vi "Main.vi"() -> ()   [LabVIEW 2016, in "Utilities.lvlib" / "Joystick.lvlib"]
uses:
  Joystick/Joystick.lvlib
  Joystick/Controls/Speed Scale.ctl
  Joystick/Controls/Up.ctl
  Joystick/Controls/Right.ctl
  Joystick/Controls/Left.ctl
  Joystick/Controls/Down.ctl
  Drivers/Agilis/AgilisCmdLib Refnum.ctl
  Drivers/Agilis/Jog Mode.ctl
  Support VIs/Message Queue/Enqueue Message (Multiple).vi
  Support VIs/Message Queue/Enqueue Message (Single).vi
  Support VIs/Message Queue/Message Queue.lvlib
  Drivers/Agilis/Agilis.lvlib
  C:/Users/MyUser/Desktop/Trace Grabber/Drivers/Agilis/AgilisCmdLib.dll
  Drivers/Agilis/AgilisCmdLib.dll
panel:
  in  "Z":cluster{"Z-":T1, "Z+":T2}
  in  "XY":cluster{"Y+":T3, "X+":T2, "X-":T1, "Y-":T4}
  in  "Speed":T5 scale=1.0..4.0
  out "Z steps":i32
  out "Y Steps":i32
  out "X steps":i32
  # "X"
  # "steps"
  # "Y"
  # "steps"
  # "Z"
  # "steps"
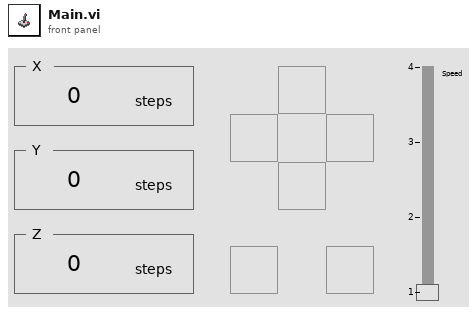
[diagram p1: front panel]
types:
  T1 = typedef "Utilities.lvlib/Joystick.lvlib/Left.ctl" = bool
  T2 = typedef "Utilities.lvlib/Joystick.lvlib/Right.ctl" = bool
  T3 = typedef "Utilities.lvlib/Joystick.lvlib/Up.ctl" = bool
  T4 = typedef "Utilities.lvlib/Joystick.lvlib/Down.ctl" = bool
  T5 = typedef "Utilities.lvlib/Joystick.lvlib/Speed Scale.ctl" = i32
  T6 = typedef "Drivers.lvlib/Agilis.lvlib/AgilisCmdLib Refnum.ctl" = refnum<k24>
  T7 = cluster{"Handle":T6, "Speed Option":i32, "Active Axis Index":i32, "Active Axis":cluster{"Channel":i32, "Axis":i32}}
  T8 = typedef "Drivers.lvlib/Agilis.lvlib/Jog Mode.ctl" = i32
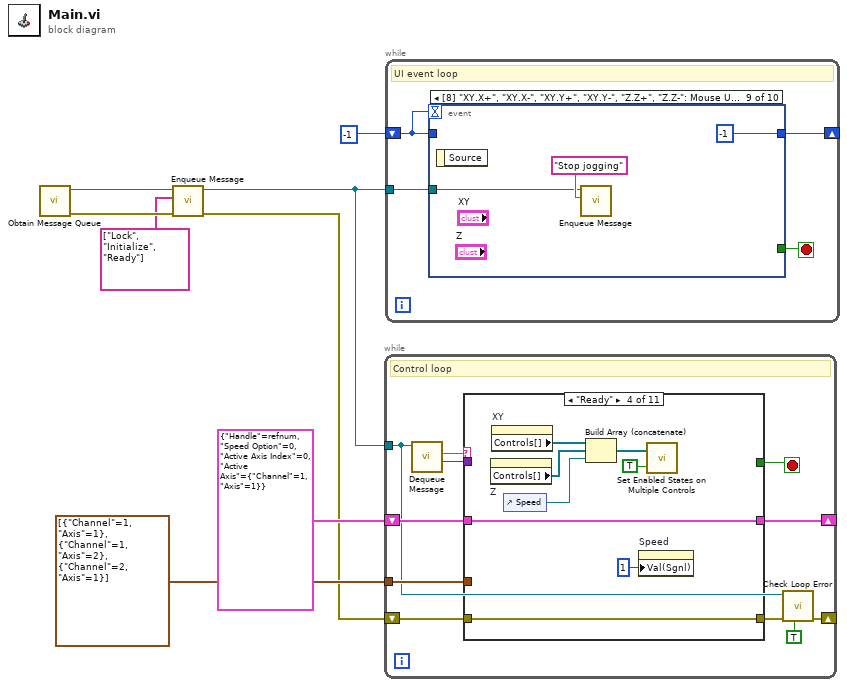
[diagram p0: block diagram]
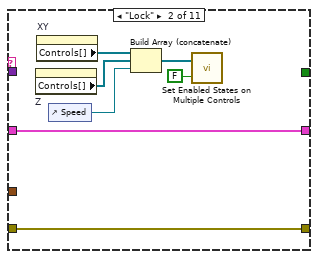
[diagram p3: hidden frame]
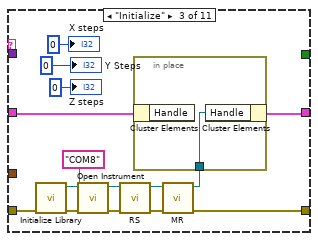
[diagram p4: hidden frame]
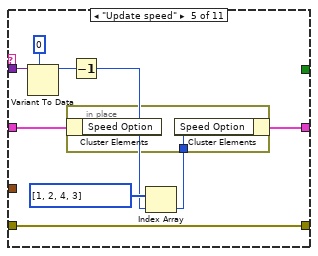
[diagram p5: hidden frame]
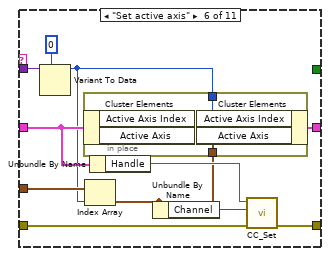
[diagram p6: hidden frame]
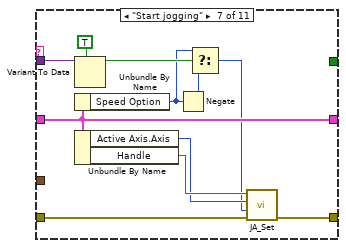
[diagram p7: hidden frame]
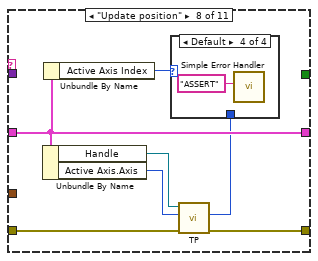
[diagram p8: hidden frame]
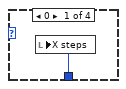
[diagram p9: hidden frame]
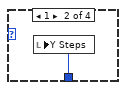
[diagram p10: hidden frame]
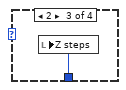
[diagram p11: hidden frame]
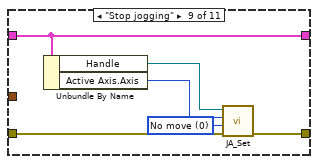
[diagram p12: hidden frame]
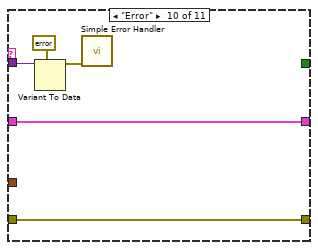
[diagram p13: hidden frame]
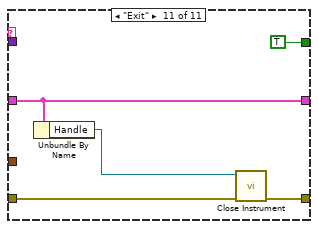
[diagram p14: hidden frame]
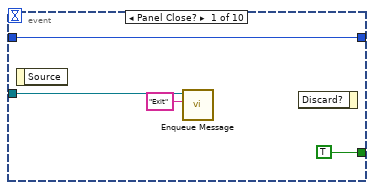
[diagram p15: hidden frame]
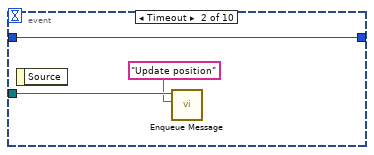
[diagram p16: hidden frame]
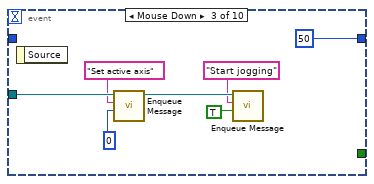
[diagram p17: hidden frame]
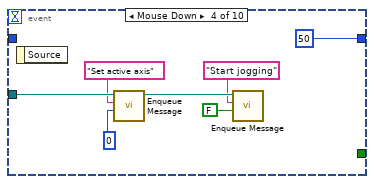
[diagram p18: hidden frame]
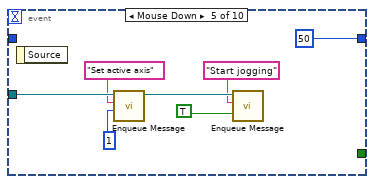
[diagram p19: hidden frame]
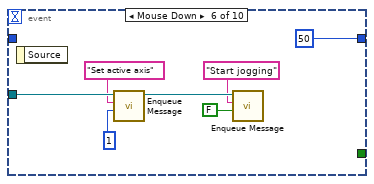
[diagram p20: hidden frame]
diagram:
  n1 = call "Obtain Message Queue.vi"() -> ("error out"=w7:errorcluster, "Message Queue out"=w8:refnum<queue>)  [unwired: 10 in]
  n2 = call-poly "Enqueue Message.vi"("error in (no error)"=w7, "States"=string[] ["Lock", "Initialize", "Ready"], "Message Queue in"=w8) -> ("error out"=w3:errorcluster, "Message Queue out"=w6:refnum<queue>)  [unwired: 7 in]
  n3 = while {
    tunnel: w6 -> [w10]
    tunnel: cluster{"Channel":i32, "Axis":i32}[] [{"Channel"=1, "Axis"=1}, {"Channel"=1, "Axis"=2}, {"Channel"=2, "Axis"=1}] -> [w18]
    shift-right: [w16] -> _
    shift-left: T7 {"Handle"=refnum, "Speed Option"=0, "Active Axis Index"=0, "Active Axis"={"Channel"=1, "Axis"=1}} -> [w15]
    shift-right: [w12] -> _
    shift-left: w3 -> [w14]
    stop <- w9 stop-if-true
    # "Control loop"
    n4 = call "Dequeue Message.vi"("Message Queue in"=w10) -> ("Data"=w17:variant, "State"=w19:string)  [unwired: 7 in, 2 out]
    n5 = case shown="\"Ready\"" w19 {
      tunnel: w18 -> [_ _ _ _ _ w70 _ _ _ _ _]
      tunnel: w15 -> [w21 w28 w40 w52 w57 w69 w81 w89 w103 w108 w113]
      tunnel: w17 -> [_ _ _ _ w60 w73 w86 _ _ w107 _]
      tunnel: [w21 w28 w39 w52 w56 w71 w81 w89 w103 w108 w113] -> w16
      tunnel: w14 -> [w20 w27 w38 w51 w53 w67 w79 w93 w99 w104 w111]
      tunnel: [w20 w27 w33 w51 w53 w66 w80 w92 w98 w104 w110] -> w13
      tunnel: [_ _ _ _ _ _ _ _ _ _ TRUE] -> w9
      frame Default {
      }
      frame "Lock" {
        n6 = property on="Z" class="Clust (strict)"() -> ("Controls[]"=w25:refnum<vi>[])  [unwired: 2 in, 2 out]
        n7 = property on="XY" class="Clust (strict)"() -> ("Controls[]"=w26:refnum<vi>[])  [unwired: 2 in, 2 out]
        n8 = control-ref of="Speed"() -> (w23:refnum<vi>)
        n9 = Build Array (concatenate)(w26, w25, w23) -> (w24:refnum<vi>[])
        n10 = call "Set Enabled States on Multiple Controls.vi"("Enable?"=FALSE, "Control Refnums"=w24) -> ()  [unwired: 1 in]
      }
      frame "Initialize" {
        n11 = call "Initialize Library.vi"("error in (no error)"=w38) -> ("error out"=w37:errorcluster, "Agilis out"=w36:T6)  [unwired: 9 in]
        n12 = call "Open Instrument.vi"("error in (no error)"=w37, "Device Key"="COM8", "Agilis in"=w36) -> ("error out"=w30:errorcluster, "Agilis out"=w32:T6)  [unwired: 7 in]
        n13 = call "RS.vi"("error in (no error)"=w30, "Agilis in"=w32) -> ("error out"=w29:errorcluster, "Agilis out"=w31:T6)  [unwired: 8 in]
        n14 = call "MR.vi"("error in (no error)"=w29, "Agilis in"=w31) -> ("error out"=w33:errorcluster, "Agilis out"=w34:T6)  [unwired: 8 in]
        n15 = in-place {
          in-place-border: w34 -> [w44]
          n16 = in-place-cluster #1(w40) -> ()  [unwired: 1 out]
          n17 = in-place-cluster #1("Handle"=w44) -> (w39:T7)
        }
        "X steps" <- 0 ("X steps")
        "Y Steps" <- 0 ("Y Steps")
        "Z steps" <- 0 ("Z steps")
      }
      frame "Ready" {
        n18 = property on="Z" class="Clust (strict)"() -> ("Controls[]"=w49:refnum<vi>[])  [unwired: 2 in, 2 out]
        n19 = property on="XY" class="Clust (strict)"() -> ("Controls[]"=w50:refnum<vi>[])  [unwired: 2 in, 2 out]
        n20 = control-ref of="Speed"() -> (w47:refnum<vi>)
        n21 = Build Array (concatenate)(w50, w49, w47) -> (w48:refnum<vi>[])
        n22 = property on="Speed" class="Slide (strict)"("Val(Sgnl)"=T5 1 ("Value (Signaling)")) -> ()  [unwired: 2 in, 2 out]
        n23 = call "Set Enabled States on Multiple Controls.vi"("Enable?"=TRUE, "Control Refnums"=w48) -> ()  [unwired: 1 in]
      }
      frame "Update speed" {
        n24 = Variant To Data(type=0, Variant=w60) -> (data=w58:i32)  [unwired: 1 in, 1 out]
        n25 = Decrement(x=w58) -> (x-1=w54:i32)
        n26 = Index Array(array=i32[] [1, 2, 4, 3], index=w54) -> (element=w55:i32)
        n27 = in-place {
          in-place-border: w55 -> [w62]
          n28 = in-place-cluster #2(w57) -> ()  [unwired: 1 out]
          n29 = in-place-cluster #2("Speed Option"=w62) -> (w56:T7)
        }
      }
      frame "Set active axis" {
        n30 = Variant To Data(type=0, Variant=w73) -> (data=w63:i32)  [unwired: 1 in, 1 out]
        n31 = Index Array(array=w70, index=w63) -> (element=w65:cluster{"Channel":i32, "Axis":i32})
        n32 = in-place {
          in-place-border: w65 -> [w75]
          in-place-border: w63 -> [w74]
          n33 = in-place-cluster #3(w69) -> ()  [unwired: 2 out]
          n34 = in-place-cluster #3("Active Axis Index"=w74, "Active Axis"=w75) -> (w71:T7)
        }
        n35 = Unbundle By Name(w69) -> ("Handle"=w68:T6)
        n36 = Unbundle By Name(w65) -> ("Channel"=w64:i32)
        n37 = call "CC_Set.vi"("error in (no error)"=w67, "Channel Number"=w64, "Agilis in"=w68) -> ("error out"=w66:errorcluster)  [unwired: 7 in, 1 out]
      }
      frame "Start jogging" {
        n38 = Variant To Data(type=TRUE, Variant=w86) -> (data=w84:bool)  [unwired: 1 in, 1 out]
        n39 = Unbundle By Name(w81) -> ("Speed Option"=w83:i32)
        n40 = Unbundle By Name(w81) -> ("Active Axis.Axis"=w77:i32, "Handle"=w78:T6)
        n41 = Negate(x=w83) -> (-x=w82:i32)
        n42 = Select(t=w83, s=w84, f=w82) -> (s? t:f=w76:i32)
        n43 = call "JA_Set.vi"("error in (no error)"=w79, "Jog Mode"=w76, "Axis Number"=w77, "Agilis in"=w78) -> ("error out"=w80:errorcluster)  [unwired: 6 in, 1 out]
      }
      frame "Update position" {
        n44 = Unbundle By Name(w89) -> ("Handle"=w91:T6, "Active Axis.Axis"=w90:i32)
        n45 = Unbundle By Name(w89) -> ("Active Axis Index"=w88:i32)
        n46 = call "TP.vi"("error in (no error)"=w93, "Axis Number"=w90, "Agilis in"=w91) -> ("error out"=w92:errorcluster, "Accumulated Steps"=w87:i32)  [unwired: 6 in, 1 out]
        n47 = case shown="Default" w88 {
          tunnel: w87 -> [w94 w95 w96 _]
          frame 0 {
            n48 = local write "X steps"(w94) -> ()
          }
          frame 1 {
            n49 = local write "Y Steps"(w95) -> ()
          }
          frame 2 {
            n50 = local write "Z steps"(w96) -> ()
          }
          frame Default {
            n51 = call <vilib>:"Simple Error Handler.vi"("error source (\" \")"="ASSERT" ("error source (\" \")")) -> ()  [unwired: 4 in, 5 out]
          }
        }
      }
      frame "Stop jogging" {
        w100 = T8 0 items=["-666 steps/s"=-4, "-1700 steps/s"=-3, "-100 steps/s"=-2, "-5 steps/s"=-1, "No move"=0, "+5 steps/s"=1, "+100 steps/s"=2, "+1700 steps/s"=3, "+666 steps/s"=4] ("Jog Mode")
        n52 = Unbundle By Name(w103) -> ("Handle"=w102:T6, "Active Axis.Axis"=w101:i32)
        n53 = call "JA_Set.vi"("error in (no error)"=w99, "Jog Mode"=w100, "Axis Number"=w101, "Agilis in"=w102) -> ("error out"=w98:errorcluster)  [unwired: 6 in, 1 out]
      }
      frame "Error" {
        n54 = Variant To Data(type=errorcluster {"status"=FALSE, "code"=0, "source"=""} ("error constant"), Variant=w107) -> (data=w105:errorcluster)  [unwired: 1 in, 1 out]
        n55 = call <vilib>:"Simple Error Handler.vi"("error in (no error)"=w105) -> ()  [unwired: 4 in, 5 out]
      }
      frame "Exit" {
        n56 = Unbundle By Name(w113) -> ("Handle"=w112:T6)
        n57 = call "Close Instrument.vi"("error in (no error)"=w111, "Agilis in"=w112) -> ("error out"=w110:errorcluster)  [unwired: 9 in]
      }
    }
    n58 = call "Check Loop Error.vi"("Exit on Error?"=TRUE, "error in (no error)"=w13, "Message Queue in"=w10) -> ("error out"=w12:errorcluster)  [unwired: 6 in, 2 out]
  }
  n59 = while {
    tunnel: w6 -> [w117]
    shift-right: [w116] -> _
    shift-left: -1 -> [w115]
    stop <- w114 stop-if-true
    # "UI event loop"
    n60 = event shown="[8] \"XY.X+\", \"XY.X-\", \"XY.Y+\", \"XY.Y-\", \"Z.Z+\", \"Z.Z-\": Mouse Up" {
      selector: _ -> [_ _ _ _ _ _ _ _ _ _]
      dyn-events: _ -> [_ _ _ _ _ _ _ _ _ _]
      timeout: w115 -> [_ _ _ _ _ _ _ _ _ _]
      tunnel: w117 -> [w119 w124 w131 w138 w145 w152 w159 w166 w167 w173]
      tunnel: [w121 w122 50 50 50 50 50 50 -1 w170] -> w116
      tunnel: w115 -> [w121 w122 _ _ _ _ _ _ _ w170]
      tunnel: [TRUE _ _ _ _ _ _ _ _ _] -> w114
      event Panel Close? {
        n61 = event-data() -> ()  [unwired: 1 in, 1 out]
        n62 = call-poly "Enqueue Message.vi"("State"="Exit", "Message Queue in"=w119) -> ()  [unwired: 8 in, 2 out]
        n63 = event-data() -> ()  [unwired: 2 in, 1 out]
      }
      event Timeout {
        n64 = event-data() -> ()  [unwired: 1 in, 1 out]
        n65 = call-poly "Enqueue Message.vi"("State"="Update position", "Message Queue in"=w124) -> ()  [unwired: 8 in, 2 out]
      }
      event Mouse Down {
        n66 = event-data() -> ()  [unwired: 1 in, 1 out]
        n67 = call-poly "Enqueue Message.vi"("Data"=0, "State"="Set active axis", "Message Queue in"=w131) -> ("Message Queue out"=w128:refnum<queue>)  [unwired: 7 in, 1 out]
        n68 = call-poly "Enqueue Message.vi"("Data"=TRUE, "State"="Start jogging", "Message Queue in"=w128) -> ()  [unwired: 7 in, 2 out]
      }
      event Mouse Down {
        n69 = event-data() -> ()  [unwired: 1 in, 1 out]
        n70 = call-poly "Enqueue Message.vi"("Data"=0, "State"="Set active axis", "Message Queue in"=w138) -> ("Message Queue out"=w135:refnum<queue>)  [unwired: 7 in, 1 out]
        n71 = call-poly "Enqueue Message.vi"("Data"=FALSE, "State"="Start jogging", "Message Queue in"=w135) -> ()  [unwired: 7 in, 2 out]
      }
      event Mouse Down {
        n72 = event-data() -> ()  [unwired: 1 in, 1 out]
        n73 = call-poly "Enqueue Message.vi"("Data"=1, "State"="Set active axis", "Message Queue in"=w145) -> ("Message Queue out"=w142:refnum<queue>)  [unwired: 7 in, 1 out]
        n74 = call-poly "Enqueue Message.vi"("Data"=TRUE, "State"="Start jogging", "Message Queue in"=w142) -> ()  [unwired: 7 in, 2 out]
      }
      event Mouse Down {
        n75 = event-data() -> ()  [unwired: 1 in, 1 out]
        n76 = call-poly "Enqueue Message.vi"("Data"=1, "State"="Set active axis", "Message Queue in"=w152) -> ("Message Queue out"=w149:refnum<queue>)  [unwired: 7 in, 1 out]
        n77 = call-poly "Enqueue Message.vi"("Data"=FALSE, "State"="Start jogging", "Message Queue in"=w149) -> ()  [unwired: 7 in, 2 out]
      }
      event Mouse Down {
        n78 = event-data() -> ()  [unwired: 1 in, 1 out]
        n79 = call-poly "Enqueue Message.vi"("Data"=2, "State"="Set active axis", "Message Queue in"=w159) -> ("Message Queue out"=w156:refnum<queue>)  [unwired: 7 in, 1 out]
        n80 = call-poly "Enqueue Message.vi"("Data"=TRUE, "State"="Start jogging", "Message Queue in"=w156) -> ()  [unwired: 7 in, 2 out]
      }
      event Mouse Down {
        n81 = event-data() -> ()  [unwired: 1 in, 1 out]
        n82 = call-poly "Enqueue Message.vi"("Data"=2, "State"="Set active axis", "Message Queue in"=w166) -> ("Message Queue out"=w163:refnum<queue>)  [unwired: 7 in, 1 out]
        n83 = call-poly "Enqueue Message.vi"("Data"=FALSE, "State"="Start jogging", "Message Queue in"=w163) -> ()  [unwired: 7 in, 2 out]
      }
      event Mouse Up {
        n84 = event-data() -> ()  [unwired: 1 in, 1 out]
        n85 = call-poly "Enqueue Message.vi"("State"="Stop jogging", "Message Queue in"=w167) -> ()  [unwired: 8 in, 2 out]
      }
      event Value Change {
        n86 = event-data() -> ()  [unwired: 1 in, 1 out]
        n87 = call-poly "Enqueue Message.vi"("Data"="Speed", "State"="Update speed", "Message Queue in"=w173) -> ()  [unwired: 7 in, 2 out]
      }
    }
  }
